vi "Is Manual Mode.vi"(8 "error in (no error)":errorcluster) -> (0 "error out":errorcluster, 1 "Manual Mode?":bool)   [LabVIEW 2015, in "cRIO-Carbondioxide.lvlib" / "cRIO-CO2.lvlib" / "cRIO-CO2.lvclass"]
uses:
  cRIO-CO2.lvclass
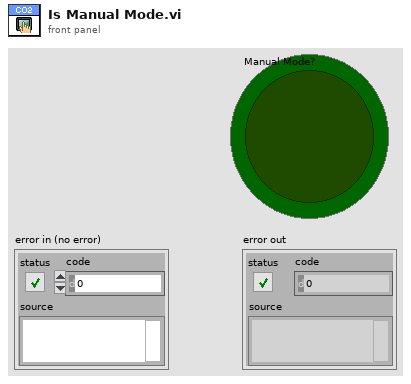
[diagram p1: front panel]
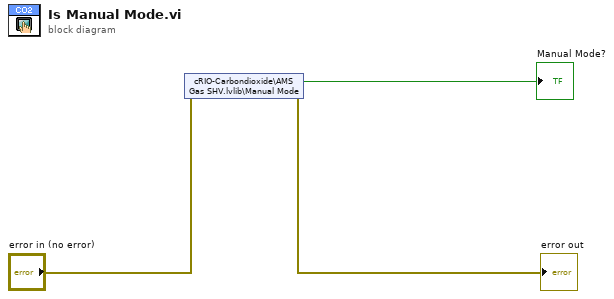
[diagram p0: block diagram]
diagram:
  n1 = shared-variable "cRIO-Carbondioxide\\AMS Gas SHV.lvlib\\Manual Mode"(error in="error in (no error)") -> (→"Manual Mode?":bool, error out=→"error out":errorcluster)
